vi "物体检测.vi"() -> ()   [LabVIEW 2020]
panel:
  in  "停止":bool
  out "Image":T1(plugin-control)
  out "Number of Objects":i32
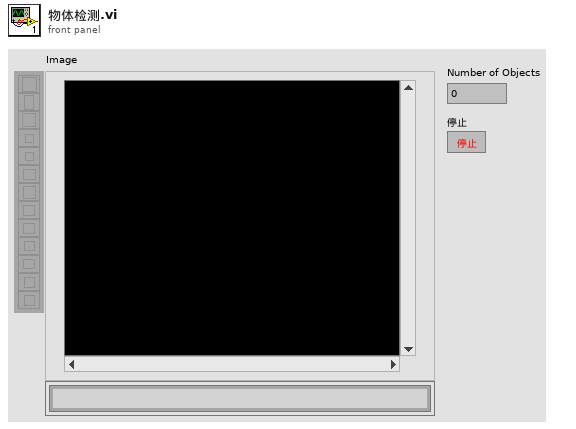
[diagram p1: front panel]
types:
  T1 = typedef "IMAQ Image.ctl" = refnum<image>
  T2 = cluster{"Objects":u16, "Threshold":i32, "Reject Border":bool, "Fill Holes":bool, "Min Object Size":bool, "Min Size":i32, "Max Object Size":bool, "Max Size":i32, "Show Search Area":bool, "Show Center":bool, "Show Bounding Box":bool}
  T3 = typedef "Image Type" = u32
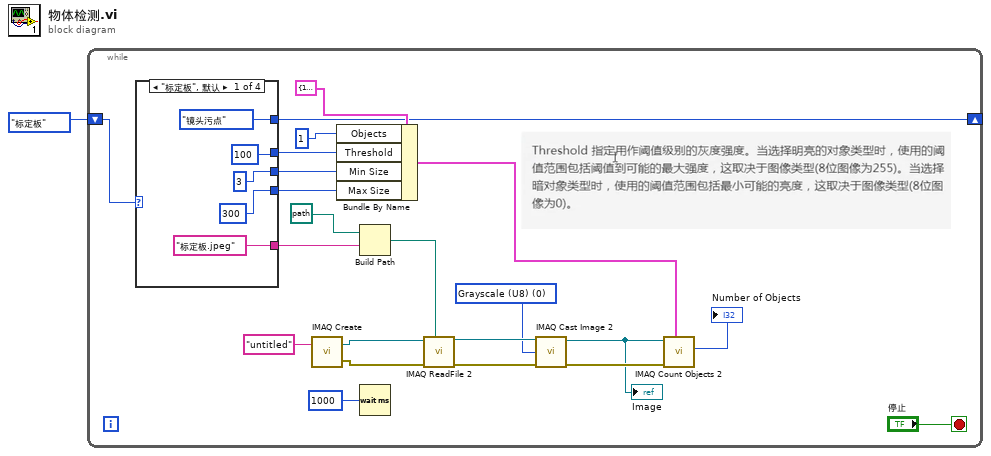
[diagram p0: block diagram]
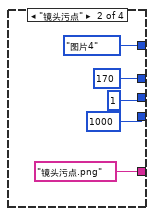
[diagram p2: hidden frame]
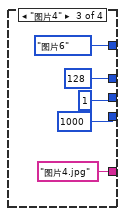
[diagram p3: hidden frame]
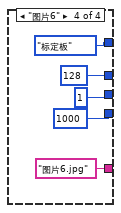
[diagram p4: hidden frame]
diagram:
  n1 = while {
    shift-right: [w4] -> _
    shift-left: enum16{"标定板", "镜头污点", "图片4", "图片6"}."标定板" ("枚举") -> [w5]
    stop <- "停止" stop-if-true
    w18 = T3 0 items=["Grayscale (U8)", "Grayscale (I16)", "Grayscale (SGL)", "Complex (CSG)", "RGB (U32)", "HSL (U32)", "RGB (U64)", "Grayscale (U16)"] ("Image Type")
    n2 = case shown="\"标定板\", 默认" w5 {
      tunnel: ["标定板.jpeg" "镜头污点.png" "图片4.jpg" "图片6.jpg"] -> w13
      tunnel: [100 170 128 128] -> w12
      tunnel: [3 1 1 1] -> w11
      tunnel: [300 1000 1000 1000] -> w10
      tunnel: [enum16{"标定板", "镜头污点", "图片4", "图片6"}."镜头污点" ("枚举") enum16{"标定板", "镜头污点", "图片4", "图片6"}."图片4" ("枚举") enum16{"标定板", "镜头污点", "图片4", "图片6"}."图片6" ("枚举") enum16{"标定板", "镜头污点", "图片4", "图片6"}."标定板" ("枚举")] -> w4
      frame "标定板", Default {
      }
      frame "镜头污点" {
      }
      frame "图片4" {
      }
      frame "图片6" {
      }
    }
    n3 = call "IMAQ Create"("Image Name"="untitled") -> ("New Image"=w21:T1, "error out"=w22:errorcluster)  [unwired: 4 in]
    n4 = Bundle By Name(cluster=T2 {"Objects"=1, "Threshold"=100, "Reject Border"=FALSE, "Fill Holes"=FALSE, "Min Object Size"=TRUE, "Min Size"=3, "Max Object Size"=TRUE, "Max Size"=300, "Show Search Area"=FALSE, "Show Center"=TRUE, "Show Bounding Box"=TRUE} ("Settings"), "Objects"=u16 1, "Threshold"=w12, "Min Size"=w11, "Max Size"=w10) -> (w8:T2)
    n5 = Build Path(base path=path "E:/朱晨辉/个人资料/01-计算机编程/00-上位机开发/02-基础知识/09-基于VISION的图像采集V2020/06-物体检测/TestFiles", name or relative path=w13) -> (appended path=w14:path)
    n6 = Wait (ms)(milliseconds to wait=u32 1000 ("等待时间（毫秒）")) -> ()  [unwired: 1 out]
    n7 = call "IMAQ ReadFile 2"("File Path"=w14, "error in (no error)"=w22, "Image"=w21) -> ("error out"=w19:errorcluster, "Image Out"=w20:T1)  [unwired: 4 in, 3 out]
    n8 = call "IMAQ Cast Image 2"("Image Src"=w20, "Image Type"=w18, "error in (no error)"=w19) -> ("Image Dst Out"=w15:T1, "error out"=w17:errorcluster)  [unwired: 11 in]
    "Image" <- w15
    n9 = call "IMAQ Count Objects 2"("Settings"=w8, "error in (no error)"=w17, "Image"=w15) -> ("Number of Objects"=→"Number of Objects":i32)  [unwired: 4 in, 4 out]
  }
